vi "Match Regular Expression_Execute.vi"(0 "input string":string, 1 "ignore case? (F)":bool, 2 "multiline? (F)":bool, 5 "regular expression":string, 9 "offset (0)":i32, 11 "error in (no error)":errorcluster) -> (4 "before match":string, 6 "whole match":string, 8 "after match":string, 10 "whole match offset":i32, 14 "matched substrings":string[](array[string]), 15 "error out":errorcluster)   [LabVIEW 2017]
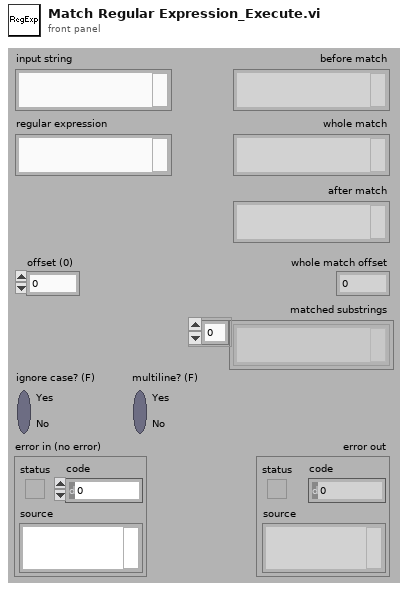
[diagram p1: front panel]
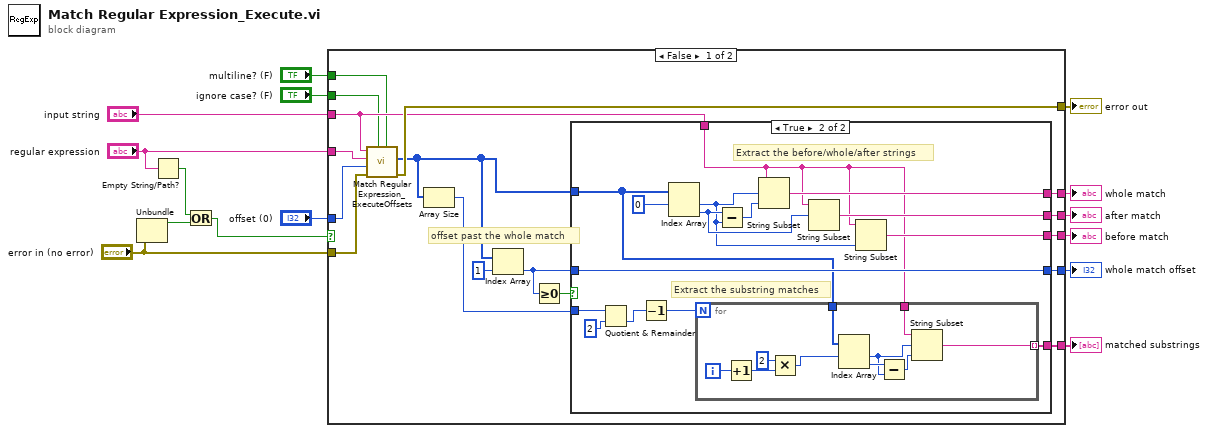
[diagram p0: block diagram]
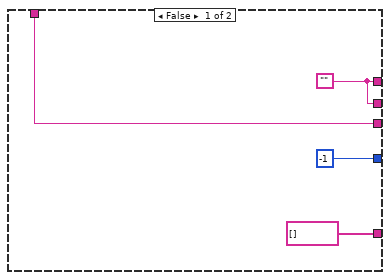
[diagram p2: hidden frame]
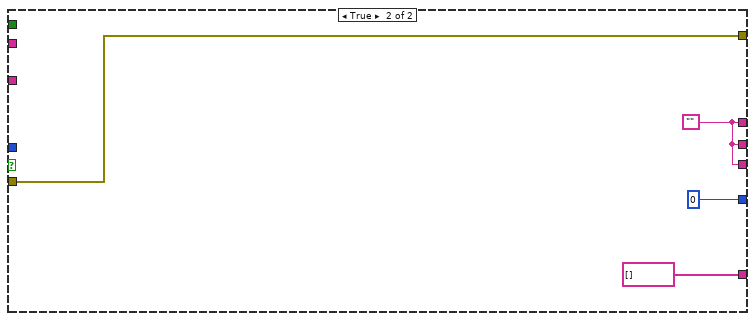
[diagram p3: hidden frame]
diagram:
  n1 = Unbundle("error in (no error)") -> ("status"=w4:bool)  [unwired: 2 out]
  n2 = Empty String/Path?(string/path="regular expression") -> (empty?=w1:bool)
  n3 = Or(x=w1, y=w4) -> (x .or. y?=w3:bool)
  n4 = case shown="False" w3 {
    tunnel: [w32 string[] []] -> w15
    tunnel: "input string" -> [w22 _]
    tunnel: [w25 w62] -> w14
    tunnel: [w30 w63] -> w13
    tunnel: [w26 0] -> w12
    tunnel: "multiline? (F)" -> [w17 _]
    tunnel: "ignore case? (F)" -> [w18 _]
    tunnel: "offset (0)" -> [w23 _]
    tunnel: "regular expression" -> [w21 _]
    tunnel: [w20 w63] -> w8
    tunnel: [w19 w63] -> w7
    tunnel: "error in (no error)" -> [w16 w62]
    frame False {
      # "offset past the whole match"
      n5 = call <vilib>:"Match Regular Expression_ExecuteOffsets.vi"("multiline? (F)"=w17, "ignore case? (F)"=w18, "error in (no error)"=w16, "offset (0)"=w23, "regular expression"=w21, "string"=w22) -> ("error out"=w25:errorcluster, "offsets"=w24:i32[])  [unwired: 4 in]
      n6 = Array Size(array=w24) -> (size(s)=w29:i32)
      n7 = Index Array(array=w24, index=1) -> (element=w27:i32)
      n8 = Greater Or Equal To 0?(x=w27) -> (x >= 0?=w28:bool)
      n9 = case shown="True" w28 {
        tunnel: [string[] [] w51] -> w32
        tunnel: w22 -> [w33 w41]
        tunnel: [w34 w48] -> w30
        tunnel: w24 -> [_ w46]
        tunnel: w29 -> [_ w40]
        tunnel: [-1 w47] -> w26
        tunnel: w27 -> [_ w47]
        tunnel: [w34 w43] -> w20
        tunnel: [w33 w42] -> w19
        frame False {
          w34 = ""
        }
        frame True {
          # "Extract the before/whole/after strings"
          # "Extract the substring matches"
          n10 = Quotient & Remainder(x=w40, y=2) -> (floor(x/y)=w38:i32)  [unwired: 1 out]
          n11 = Decrement(x=w38) -> (x-1=w37:i32)
          n12 = Index Array(array=w46, index #1=0 ("index")) -> (element #1=w44:i32, element #2=w45:i32)  [unwired: 1 in]
          n13 = for {
            N: w37 -> [_]
            tunnel: w46 -> [w55]
            tunnel: w41 -> [w56]
            tunnel: [w52] -> w51 mode=indexing
            i -> [w53]
            n14 = Increment(x=w53) -> (x+1=w61:i32)
            n15 = Multiply(x=2, y=w61) -> (x*y=w54:i32)
            n16 = Index Array(array=w55, index #1=w54) -> (element #1=w57:i32, element #2=w58:i32)  [unwired: 1 in]
            n17 = Subtract(x=w58, y=w57) -> (x-y=w59:i32)
            n18 = String Subset(string=w56, offset (0)=w57, length (rest)=w59) -> (substring=w52:string)
          }
          n19 = Subtract(x=w45, y=w44) -> (x-y=w49:i32)
          n20 = String Subset(string=w41, offset (0)=w44, length (rest)=w49) -> (substring=w48:string)
          n21 = String Subset(string=w41, offset (0)=w45) -> (substring=w43:string)  [unwired: 1 in]
          n22 = String Subset(string=w41, length (rest)=w44) -> (substring=w42:string)  [unwired: 1 in]
        }
      }
    }
    frame True {
      w63 = ""
    }
  }
  "error out" <- w14
  "matched substrings" <- w15
  "whole match" <- w13
  "whole match offset" <- w12
  "before match" <- w7
  "after match" <- w8
